vi "Example_DIO.vi"() -> ()   [LabVIEW 2013]
uses:
  Instance           6 19Saved   Example_DIO .vi
panel:
  in  "End Line":i32=19
  in  "Start Line":i32=16
  in  "End Line":i32=5
  in  "Start Line":i32=2
  in  "Slot":i32=4
  out "ConfigBus Out Status":errorcluster
  out "Port A Value (Hex)":i64 format="%08x"
  out "DirConfig":errorcluster
  out "ConfigBus In Status":errorcluster
  out "Bus In 0 value":i64
  out "Data => PortA\n                BusOut":i32
  out "Close Status":errorcluster
  in  "Stop Loop":bool
  out "Open Status":errorcluster
  in  "Part Number":string="SD-PXE-DIO-H0002-1G"
  # "Input Bus"
  # "Outputt Bus"
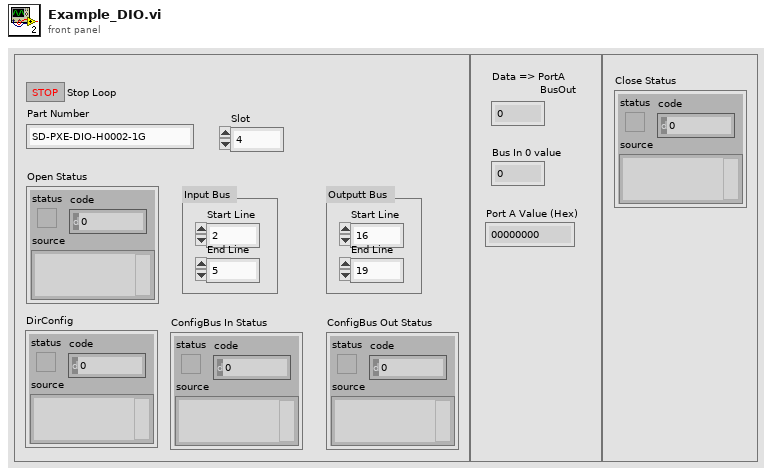
[diagram p1: front panel]
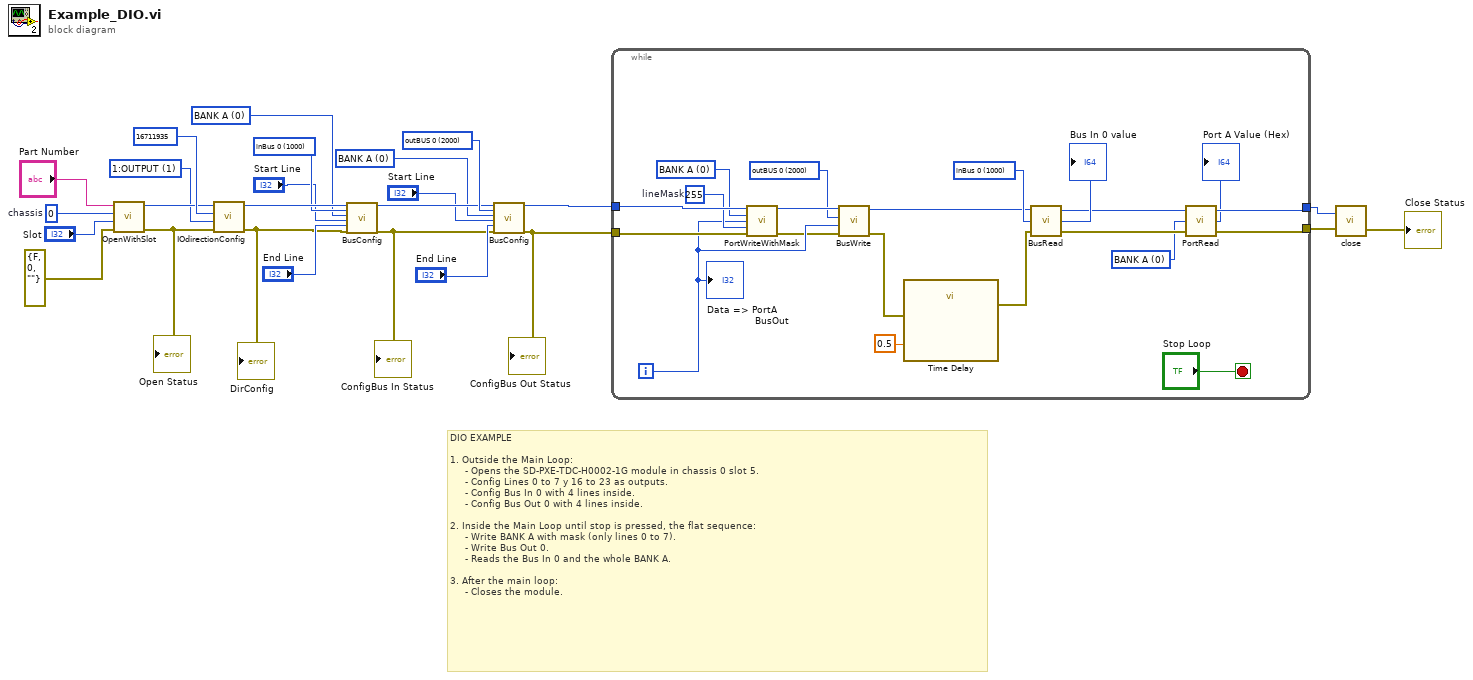
[diagram p0: block diagram]
diagram:
  w1 = 0 items=["BANK A"=0, "BANK B"=1, "BANK B:A"=3000] ("nPort")
  w2 = 0 items=["BANK A"=0, "BANK B"=1, "BANK B:A"=3000] ("nPort")
  w16 = 2000 items=["inBus 0"=1000, "outBUS 0"=2000] ("nBus")
  w17 = 1000 items=["inBus 0"=1000, "outBUS 0"=2000] ("nBus")
  w19 = u16 1 items=["0:INPUT", "1:OUTPUT"] ("direction")
  w23 = 0  # chassis
  # "DIO EXAMPLE\n\n1. Outside the Main Loop:\n     - Opens the SD-PXE-TDC-H0002-1G module in chassis 0 slot 5.\n     - Config Lines 0 to 7 y 16 to 23 as outputs.\n     - Config Bus In 0 with 4 lines inside.\n     - Config Bus Out 0 with 4 lines inside.\n\n2. Inside the Main Loop until stop is pressed, the flat sequence:\n     - Write BANK A with mask (only lines 0 to 7).\n     - Write Bus Out 0.\n     - Reads the Bus In 0 and the whole BANK A.\n\n3. After the main loop:\n     - Closes the module."
  n1 = call <vilib>:"OpenWithSlot.vi"("errorIn"=errorcluster {"status"=FALSE, "code"=0, "source"=""}, "nSlot"="Slot", "nChassis"=w23, "partNumber"="Part Number") -> ("errorOut"=w22:errorcluster, "moduleID"=w20:i32)  [unwired: 2 in]
  "Open Status" <- w22
  n2 = call <vilib>:"IOdirectionConfig.vi"("errorIn"=w22, "direction"=w19, "lineMask"=i64 16711935, "moduleID"=w20) -> ("errorOut"=w3:errorcluster, "moduleIDOut"=w18:i32)  [unwired: 2 in]
  "DirConfig" <- w3
  n3 = call <vilib>:"BusConfig.vi"("moduleID"=w18, "nBus"=w17, "port"=w2, "start"="Start Line", "end"="End Line", "errorIn"=w3) -> ("moduleIDOut"=w15:i32, "errorOut"=w4:errorcluster)  [unwired: 12 in]
  "ConfigBus In Status" <- w4
  n4 = call <vilib>:"BusConfig.vi"("moduleID"=w15, "nBus"=w16, "port"=w1, "start"="Start Line", "end"="End Line", "errorIn"=w4) -> ("moduleIDOut"=w14:i32, "errorOut"=w13:errorcluster)  [unwired: 12 in]
  "ConfigBus Out Status" <- w13
  n5 = while {
    tunnel: [w29] -> w11
    tunnel: [w28] -> w12
    tunnel: w14 -> [w41]
    tunnel: w13 -> [w39]
    i -> [w35]
    stop <- "Stop Loop" stop-if-true
    w30 = 0 items=["BANK A"=0, "BANK B"=1, "BANK B:A"=3000] ("nPort")
    w36 = 2000 items=["outBUS 0"=2000] ("nOutBus")
    w38 = i64 255  # lineMask
    w43 = 1000 items=["inBus 0"=1000] ("nInBus")
    w40 = 0 items=["BANK A"=0, "BANK B"=1, "BANK B:A"=3000] ("nPort")
    n6 = call <vilib>:"PortWriteWithMask.vi"("moduleID"=w41, "nPort"=w40, "portValue"=w35, "lineMask"=w38, "errorIn"=w39) -> ("moduleIDOut"=w37:i32, "errorOut"=w34:errorcluster)  [unwired: 9 in]
    n7 = call <vilib>:"BusWrite.vi"("errorIn"=w34, "value"=w35, "outBus"=w36, "moduleID"=w37) -> ("errorOut"=w26:errorcluster, "moduleIDOut"=w33:i32)  [unwired: 2 in]
    n8 = call "Time Delay"("error in (no error)"=w26, "Delay Time (s)"=0.5) -> ("error out"=w44:errorcluster)  [unwired: 9 in]
    n9 = call <vilib>:"BusRead.vi"("errorIn"=w44, "inBus"=w43, "moduleID"=w33) -> ("errorOut"=w31:errorcluster, "portValue"=→"Bus In 0 value":i64, "moduleIDOut"=w32:i32)
    n10 = call <vilib>:"PortRead.vi"("errorIn"=w31, "nPort"=w30, "moduleID"=w32) -> ("errorOut"=w28:errorcluster, "portValue"=→"Port A Value (Hex)":i64, "moduleIDOut"=w29:i32)
    "Data => PortA\n                BusOut" <- w35
  }
  n11 = call <vilib>:"close.vi"("errorIn"=w12, "moduleID"=w11) -> ("errorOut"=→"Close Status":errorcluster)  [unwired: 1 in]
